vi "Interpolate Color V8.vi"(2 "Size (256)":i32=256, 3 "Colors in":u8[](array[numeric])) -> (1 "Colors out":u8[](array[numeric]))   [LabVIEW 2019, in "graph_utilities.lvclass"]
uses:
  graph_utilities.lvclass
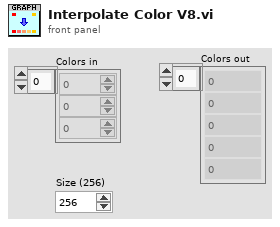
[diagram p1: front panel]
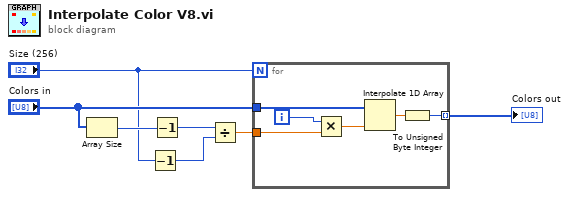
[diagram p0: block diagram]
diagram:
  n1 = Array Size(array="Colors in") -> (size(s)=w3:i32)
  n2 = Decrement(x="Size (256)") -> (x-1=w5:i32)
  n3 = Decrement(x=w3) -> (x-1=w4:i32)
  n4 = Divide(x=w4, y=w5) -> (x/y=w2:dbl)
  n5 = for {
    N: "Size (256)" -> [_]
    tunnel: "Colors in" -> [w13]
    tunnel: [w10] -> w7 mode=indexing
    tunnel: w2 -> [w8]
    i -> [w11]
    n6 = Multiply(x=w11, y=w8) -> (x*y=w9:dbl)
    n7 = Interpolate 1D Array(1:w9, 2:w13) -> (0:w12:dbl)
    n8 = To Unsigned Byte Integer(number=w12) -> (unsigned 8bit integer=w10:u8)
  }
  "Colors out" <- w7
